vi "testPresuer.vi"() -> (1 "b":dbl, 2 "k":dbl, 3 "error out":errorcluster)   [LabVIEW 2011]
uses:
  <vilib>/Utility/error.llb/DialogType.ctl
  <vilib>/DAQmx/read.llb/DAQmx Read (Analog DBL 1Chan 1Samp).vi
  <vilib>/DAQmx/create/channels.llb/DAQmx Create Channel (AI-Voltage-Basic).vi
  <vilib>/DAQmx/configure/timing.llb/DAQmx Timing (Sample Clock).vi
  <vilib>/DAQmx/miscellaneous.llb/DAQmx Fill In Error Info.vi
  <vilib>/gmath/NI_Gmath.lvlib
panel:
  in  "Tab Control 2":enum32{"Page 1", "Page 2"}(tab)
  out "线性曲线":cluster{dbl[], "Best Exponential Fit":dbl[]}[](graph)=[{[0.0, 1.0, 2.0, 3.0, 4.0, 5.0], "Best Exponential Fit"=[1.0, 2.700000047683716, 7.400000095367432, 30.0, 180.0, 400.0]}, {[0.0, 1.0, 2.0, 3.0, 4.0, 5.0], "Best Exponential Fit"=[-78.59047614960443, -5.747619013559245, 67.09523812248594, 139.93809525853112, 212.7809523945763, 285.6238095306215]}]
  out "表达式:":string="y = -78.590E+0 + 72.843E+0x"
  in  "计算":bool
  in  "退出":bool
  in  "x":dbl format="%0.2f"
  out "y":dbl format="%0.2f"
  in  "x":string[][](array[string])
  in  "Tab Control":enum32{"采集数据", "Page 2"}(tab)
  in  "x 值":dbl[](array[numeric])
  in  "采集":bool
  in  "Physical Channel":tag="Dev1/ai0" caption="物理通道"
  in  "Rate":dbl=1.0 caption="采样率 (Hz)" format="%0.2f"
  in  "Minimum Value":dbl=-10.0 caption="最小值" format="%0.2f"
  in  "Maximum Value":dbl=10.0 caption="最大值" format="%0.2f"
  out "数据曲线":dbl(graph)
  in  "精度":dbl=0.5
  in  "特征点分辨率":i32=10
  in  "试验结果y值":dbl[](array[numeric])
  in  "手动设置点":bool=TRUE
  in  "采集数据":dbl[](array[numeric])
  # "传感器参数校准"
  # "y"
  # "y=kx+b"
  # "y="
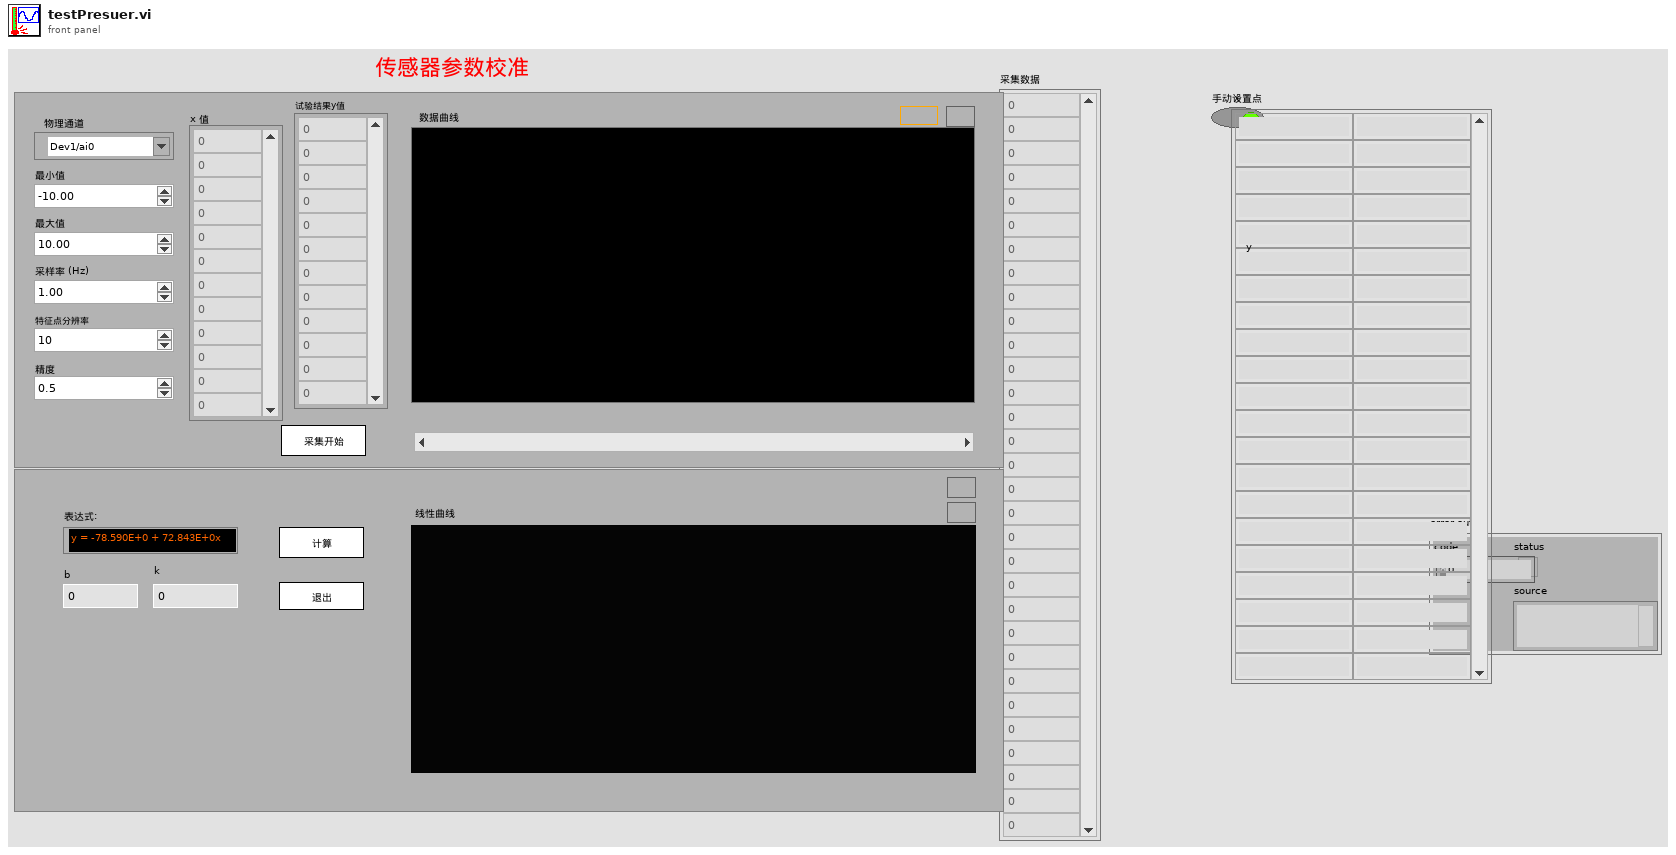
[diagram p1: front panel]
types:
  T1 = enum16{"初始化", "采集开始", "采集", "采集结束", "算出特征点", "转线性的公式", "计算", "退出"}
  T2 = typedef "DialogType.ctl" = u16
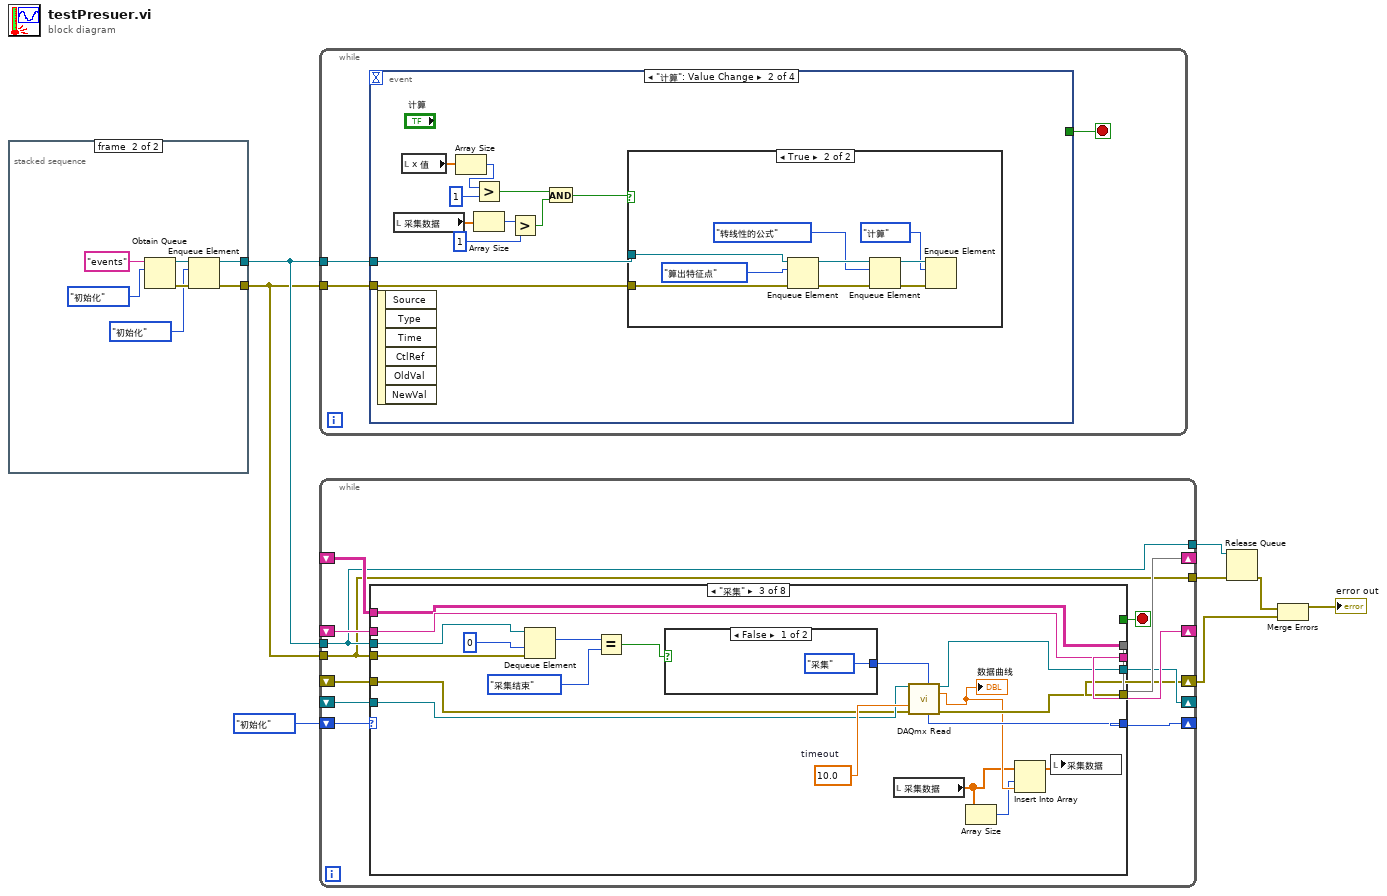
[diagram p0: block diagram]
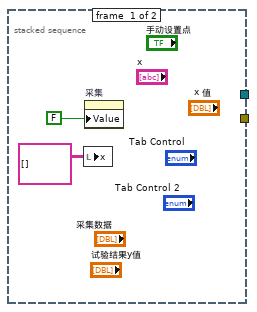
[diagram p2: hidden frame]
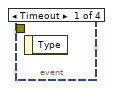
[diagram p3: hidden frame]
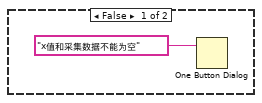
[diagram p4: hidden frame]
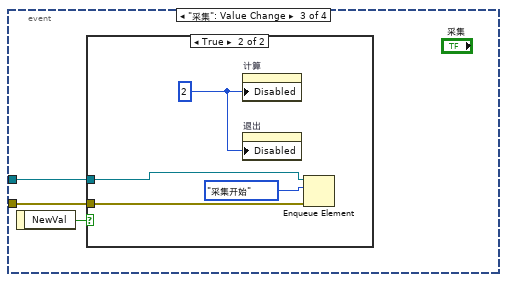
[diagram p5: hidden frame]
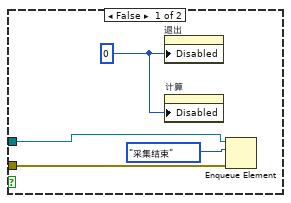
[diagram p6: hidden frame]
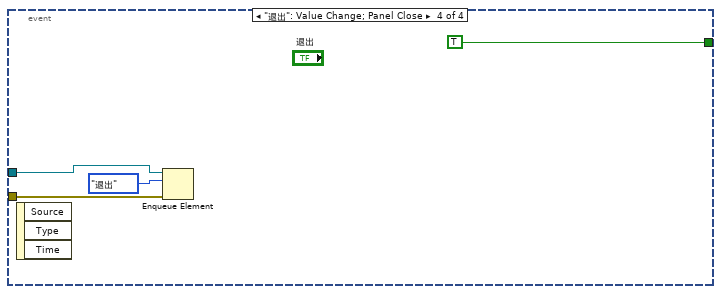
[diagram p7: hidden frame]
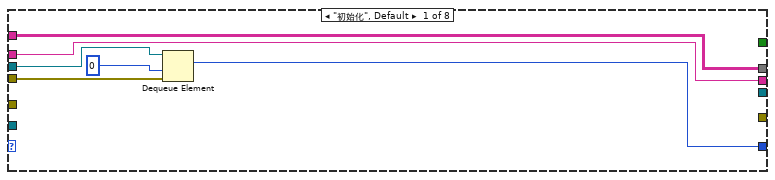
[diagram p8: hidden frame]
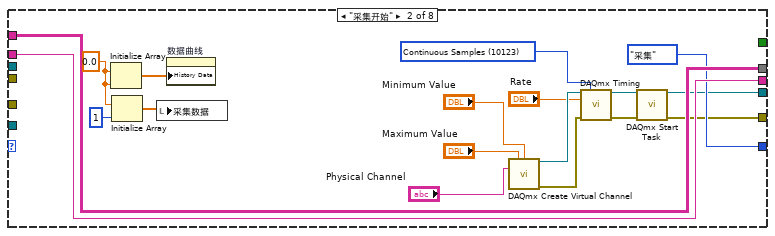
[diagram p9: hidden frame]
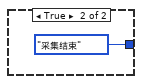
[diagram p10: hidden frame]
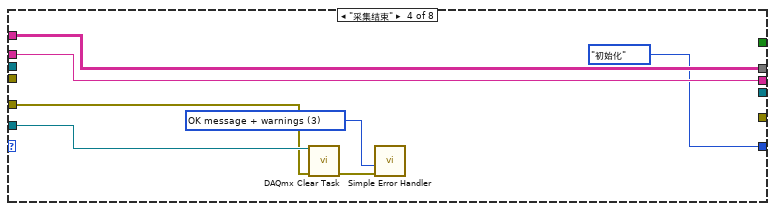
[diagram p11: hidden frame]
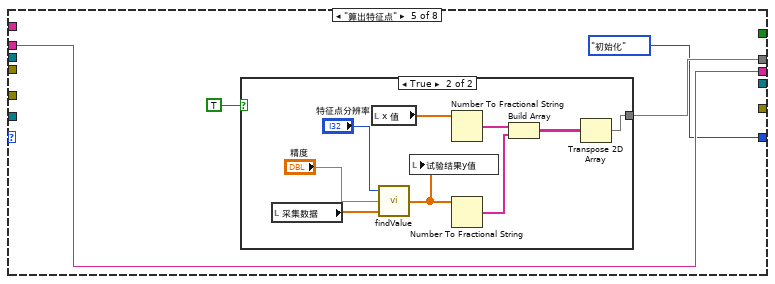
[diagram p12: hidden frame]
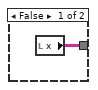
[diagram p13: hidden frame]
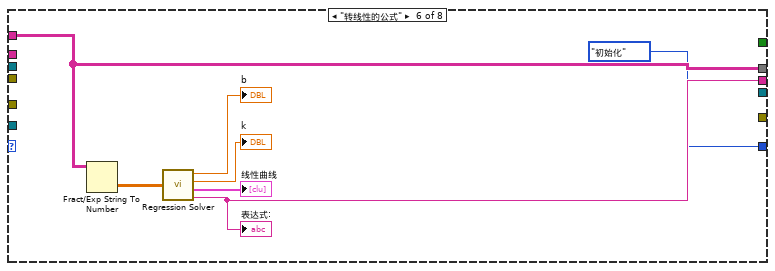
[diagram p14: hidden frame]
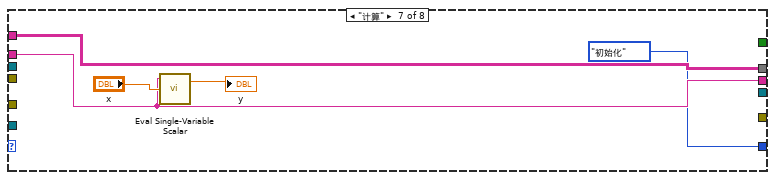
[diagram p15: hidden frame]
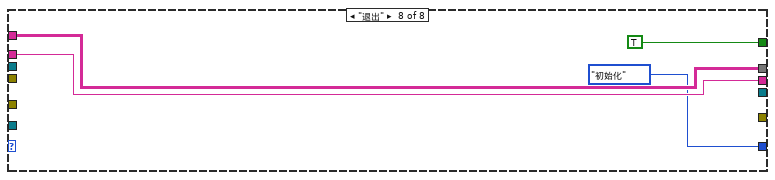
[diagram p16: hidden frame]
diagram:
  n1 = stacked-sequence {
    tunnel: [_ w14] -> w8
    tunnel: [_ w13] -> w7
    frame #0 {
      n2 = local write "x"(string[][] []) -> ()
      n3 = property on="采集" class="Bool (strict)"("Value"=FALSE ("采集")) -> ()  [unwired: 2 in, 2 out]
    }
    frame #1 {
      n4 = Obtain Queue(name (unnamed)="events", element data type=T1."初始化" ("操作")) -> (queue out=w16:refnum<queue>, error out=w15:errorcluster)  [unwired: 3 in, 1 out]
      n5 = Enqueue Element(queue=w16, element=T1."初始化" ("操作"), error in (no error)=w15) -> (queue out=w14:refnum<queue>, error out=w13:errorcluster)  [unwired: 2 out]
    }
  }
  n6 = while {
    tunnel: w8 -> [w20]
    tunnel: w7 -> [w19]
    stop <- w18 stop-if-true
    n7 = event shown="[1] \"计算\": Value Change" {
      selector: _ -> [_ _ _ _]
      dyn-events: _ -> [_ _ _ _]
      timeout: _ -> [_ _ _ _]
      tunnel: w20 -> [_ w31 w43 w55]
      tunnel: w19 -> [_ w30 w42 w54]
      tunnel: [_ _ _ TRUE] -> w18
      event Timeout {
        n8 = event-data() -> ()  [unwired: 2 out]
      }
      event "计算": Value Change {
        n9 = event-data() -> ()  [unwired: 7 out]
        n10 = local read "采集数据"() -> (w26:dbl[])
        n11 = local read "x 值"() -> (w29:dbl[])
        n12 = Array Size(array=w29) -> (size(s)=w28:i32)
        n13 = Greater?(x=w28, y=1) -> (0:w22:bool)
        n14 = Array Size(array=w26) -> (size(s)=w25:i32)
        n15 = Greater?(x=w25, y=1) -> (0:w23:bool)
        n16 = And(x=w22, y=w23) -> (x .and. y?=w21:bool)
        n17 = case shown="True" w21 {
          tunnel: w31 -> [_ w39]
          tunnel: w30 -> [_ w38]
          frame False {
            n18 = One Button Dialog(message="x值和采集数据不能为空") -> ()  [unwired: 2 out]
          }
          frame True {
            n19 = Enqueue Element(queue=w39, element=T1."算出特征点" ("操作"), error in (no error)=w38) -> (queue out=w37:refnum<queue>, error out=w36:errorcluster)  [unwired: 2 out]
            n20 = Enqueue Element(queue=w37, element=T1."转线性的公式" ("操作"), error in (no error)=w36) -> (queue out=w41:refnum<queue>, error out=w40:errorcluster)  [unwired: 2 out]
            n21 = Enqueue Element(queue=w41, element=T1."计算" ("操作"), error in (no error)=w40) -> ()  [unwired: 1 in, 3 out]
          }
        }
      }
      event "采集": Value Change {
        n22 = event-data() -> ("NewVal"=w44:bool)  [unwired: 1 out]
        n23 = case shown="True" w44 {
          tunnel: w43 -> [w48 w52]
          tunnel: w42 -> [w47 w51]
          frame False {
            w45 = u8 0 ("Disabled")
            n24 = property on="退出" class="Bool"("Disabled"=w45) -> ()  [unwired: 2 in, 2 out]
            n25 = property on="计算" class="Bool"("Disabled"=w45) -> ()  [unwired: 2 in, 2 out]
            n26 = Enqueue Element(queue=w48, element=T1."采集结束" ("操作"), error in (no error)=w47) -> ()  [unwired: 4 out]
          }
          frame True {
            w49 = u8 2 ("Disabled")
            n27 = property on="计算" class="Bool"("Disabled"=w49) -> ()  [unwired: 2 in, 2 out]
            n28 = property on="退出" class="Bool"("Disabled"=w49) -> ()  [unwired: 2 in, 2 out]
            n29 = Enqueue Element(queue=w52, element=T1."采集开始" ("操作"), error in (no error)=w51) -> ()  [unwired: 4 out]
          }
        }
      }
      event "退出": Value Change; Panel Close {
        n30 = event-data() -> ()  [unwired: 4 out]
        n31 = Enqueue Element(queue=w55, element=T1."退出" ("操作"), error in (no error)=w54) -> ()  [unwired: 4 out]
      }
    }
  }
  n32 = while {
    shift-right: [w69] -> _
    shift-left: _ -> [w68]
    shift-right: [w67] -> _
    shift-left: _ -> [w66]
    tunnel: w8 -> [w63]
    tunnel: w7 -> [w62]
    shift-right: [w61] -> _
    shift-left: T1."初始化" ("操作") -> [w65]
    tunnel: [w63] -> w6
    tunnel: [w62] -> w5
    shift-right: [w60] -> _
    shift-left: _ -> [w58]
    shift-right: [w59] -> w2
    shift-left: _ -> [w57]
    stop <- w64 stop-if-true
    n33 = case shown="\"采集\"" w65 {
      tunnel: [w75 w93 w103 w120 w124 w140 w143 w148] -> w69
      tunnel: w68 -> [w75 w93 w103 w120 _ w140 w143 w148]
      tunnel: [w74 w92 w104 w119 w123 w139 w144 w149] -> w67
      tunnel: w66 -> [w74 w92 w104 w119 w123 _ w144 w149]
      tunnel: w63 -> [w73 _ w110 _ _ _ _ _]
      tunnel: w62 -> [w72 _ w109 _ _ _ _ _]
      tunnel: [_ _ _ _ _ _ _ TRUE] -> w64
      tunnel: [w70 T1."采集" ("操作") w105 T1."初始化" ("操作") T1."初始化" ("操作") T1."初始化" ("操作") T1."初始化" ("操作") T1."初始化" ("操作")] -> w61
      tunnel: [_ w81 w99 _ _ _ _ _] -> w60
      tunnel: [_ w80 w98 _ _ _ _ _] -> w59
      tunnel: w58 -> [_ _ w101 w115 _ _ _ _]
      tunnel: w57 -> [_ _ w100 w114 _ _ _ _]
      frame "初始化", Default {
        n34 = Dequeue Element(queue=w73, timeout in ms (-1)=0, error in (no error)=w72) -> (element=w70:T1)  [unwired: 3 out]
      }
      frame "采集开始" {
        w78 = 0.0 ("element")
        w88 = 10123 items=["Finite Samples"=10178, "Continuous Samples"=10123] ("sample mode")
        n35 = Initialize Array(w78, w78) -> (w79:dbl[])
        n36 = Initialize Array(w78, 1 ("dimension size")) -> (w76:dbl[])
        n37 = local write "采集数据"(w76) -> ()
        n38 = property on="数据曲线" class="WFChart (strict)"("History Data"=w79) -> ()  [unwired: 2 in, 2 out]
        n39 = call-poly <vilib>:"DAQmx Create Virtual Channel.vi"("maximum value"="Maximum Value", "minimum value"="Minimum Value", "physical channels"="Physical Channel") -> ("task out"=w86:refnum<k21>, "error out"=w84:errorcluster)  [unwired: 6 in, 5 out]
        n40 = call-poly <vilib>:"DAQmx Timing.vi"("task/channels in"=w86, "sample mode"=w88, "rate"="Rate", "error in"=w84) -> ("task out"=w89:refnum<k21>, "error out"=w90:errorcluster)  [unwired: 3 in, 7 out]
        n41 = call <vilib>:"DAQmx Start Task.vi"("task/channels in"=w89, "error in"=w90) -> ("task out"=w81:refnum<k21>, "error out"=w80:errorcluster)  [unwired: 12 out]
      }
      frame "采集" {
        w102 = 10.0  # timeout
        n42 = Dequeue Element(queue=w110, timeout in ms (-1)=0, error in (no error)=w109) -> (element=w107:T1)  [unwired: 3 out]
        n43 = Equal?(x=w107, y=T1."采集结束" ("操作")) -> (x = y?=w106:bool)
        n44 = case shown="False" w106 {
          tunnel: [T1."采集" ("操作") T1."采集结束" ("操作")] -> w105
          frame False {
          }
          frame True {
          }
        }
        n45 = local read "采集数据"() -> (w95:dbl[])
        n46 = call-poly <vilib>:"DAQmx Read.vi"("task/channels in"=w101, "timeout"=w102, "error in"=w100) -> ("task out"=w99:refnum<k21>, "data"=w97:dbl, "error out"=w98:errorcluster)  [unwired: 1 in, 9 out]
        "数据曲线" <- w97
        n47 = Array Size(array=w95) -> (size(s)=w94:i32)
        n48 = Insert Into Array(array=w95, index=w94, new element=w97) -> (w96:dbl[])
        n49 = local write "采集数据"(w96) -> ()
      }
      frame "采集结束" {
        w117 = T2 3 items=["no dialog", "OK message", "continue or stop message", "OK message + warnings", "continue/stop + warnings"] ("type of dialog (OK msg:1)")
        n50 = call <vilib>:"DAQmx Clear Task.vi"("task in"=w115, "error in"=w114) -> ("error out"=w116:errorcluster)  [unwired: 13 out]
        n51 = call <vilib>:"Simple Error Handler.vi"("type of dialog (OK msg:1)"=w117, "error in (no error)"=w116) -> ()  [unwired: 8 out]
      }
      frame "算出特征点" {
        n52 = case shown="True" TRUE {
          tunnel: [w125 w128] -> w124
          frame False {
            n53 = local read "x"() -> (w125:string[][])
          }
          frame True {
            n54 = local read "采集数据"() -> (w127:dbl[])
            n55 = local read "x 值"() -> (w130:dbl[])
            n56 = call "findValue.vi"("采集数据"=w127, "精度"="精度", "循环点"="特征点分辨率") -> ("试验结果"=w126:dbl[])
            n57 = local write "试验结果y值"(w126) -> ()
            n58 = Number To Fractional String(number=w130) -> (F-format string=w134:string[])  [unwired: 3 out]
            n59 = Number To Fractional String(number=w126) -> (F-format string=w133:string[])  [unwired: 3 out]
            n60 = Build Array(w134, w133) -> (w129:string[][])
            n61 = Transpose 2D Array(2D array=w129) -> (transposed array=w128:string[][])
          }
        }
      }
      frame "转线性的公式" {
        n62 = Fract/Exp String To Number(string=w140) -> (number=w138:dbl[][])  [unwired: 4 out]
        n63 = call "Regression Solver.vi"("Data"=w138) -> ("b"=→"b":dbl, "k"=→"k":dbl, "Raw Data and Fitted Curve"=→"线性曲线":cluster{dbl[], "Best Exponential Fit":dbl[]}[], "Equation of Fit"=w139:string)
        "表达式:" <- w139
      }
      frame "计算" {
        n64 = call <vilib>:"Eval Single-Variable Scalar.vi"("x value"="x", "formula"=w144) -> ("y value"=→"y":dbl)  [unwired: 1 in, 1 out]
      }
      frame "退出" {
      }
    }
  }
  n65 = Release Queue(queue=w6, error in (no error)=w5) -> (error out=w3:errorcluster)  [unwired: 3 out]
  n66 = Merge Errors(w3, w2) -> (→"error out":errorcluster)
